vi "tcp connection ref.vi"(6 "init":bool, 8 "Error In":errorcluster, 10 "port (10000)":u16=10000) -> (0 "Error Out":errorcluster, 3 "tcpRef":refnum<k5>)   [LabVIEW 2016, in "mqtt.lvlib"]
uses:
  mqtt.lvlib
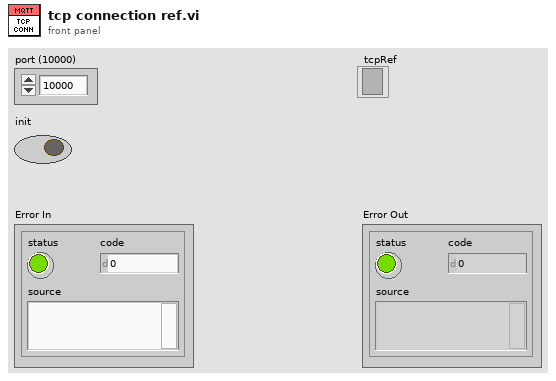
[diagram p1: front panel]
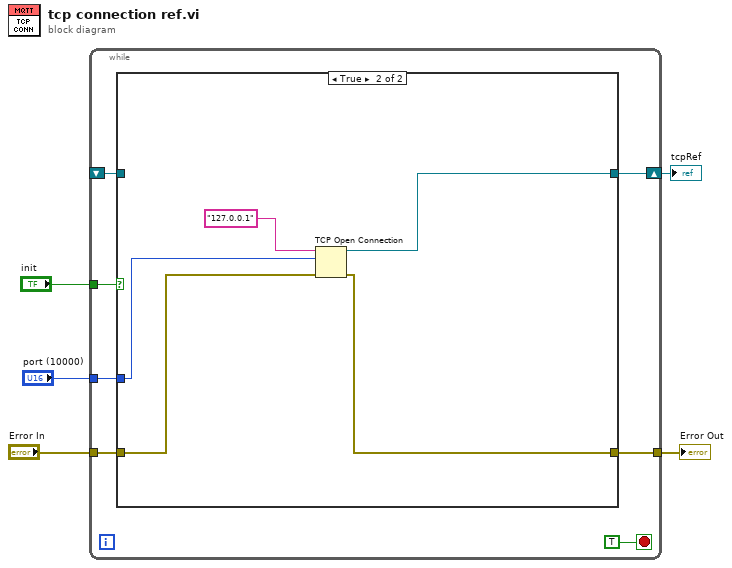
[diagram p0: block diagram]
diagram:
  n1 = while {
    tunnel: "init" -> [w11]
    tunnel: "port (10000)" -> [w10]
    shift-right: [w9] -> w1
    shift-left: _ -> [w7]
    tunnel: "Error In" -> [w8]
    tunnel: [w6] -> w2
    stop <- TRUE stop-if-true
    n2 = case shown="True" w11 {
      tunnel: w10 -> [_ w18]
      tunnel: [w14 w17] -> w9
      tunnel: w8 -> [w13 w16]
      tunnel: w7 -> [w14 _]
      tunnel: [w13 w15] -> w6
      frame False {
      }
      frame True {
        n3 = TCP Open Connection(address="127.0.0.1", remote port or service name=w18, error in (no error)=w16) -> (connection ID=w17:refnum<k5>, error out=w15:errorcluster)  [unwired: 2 in]
      }
    }
  }
  "Error Out" <- w2
  "tcpRef" <- w1
